vi "robot_focus.vi"(7 "Robot_connection":refnum<k5>, 8 "rotation_parameters":T4={"circle_radius (mm)"=6.5, "total_circle_angle (deg)"=0.0, "circle number of points"=18}, 9 "focus_parameters":T3={"Robot_vel"=0.3, "Robot_acc"=0.1, "Z-tolerance (mm)"=0.2, "Angle tolerance (deg)"=1.0, "n_frames"=1, "frame_width"=500}, 10 "Buttons":T2, 11 "img":u8[][](array[numeric])) -> (0 "wait_frames":dbl, 1 "indicators":T1, 2 "apply_config":bool, 3 "Fast_axis":bool)   [LabVIEW 2021]
panel:
  out "img_size_2":dbl
  out "img_size_1":dbl
  out "circle_state_indicator":dbl
  out "Close enough":bool
  out "angle":dbl
  in  "movement_wait_frames":dbl=5.0
  out "focus_routine_indicator":i8
  out "stepwise_angle":dbl
  in  "circle_state":i8=-2
  in  "freedrive_state":i8
  out "message_output":string
  in  "focus_routine_state":i8
  # "Robot Focus code"
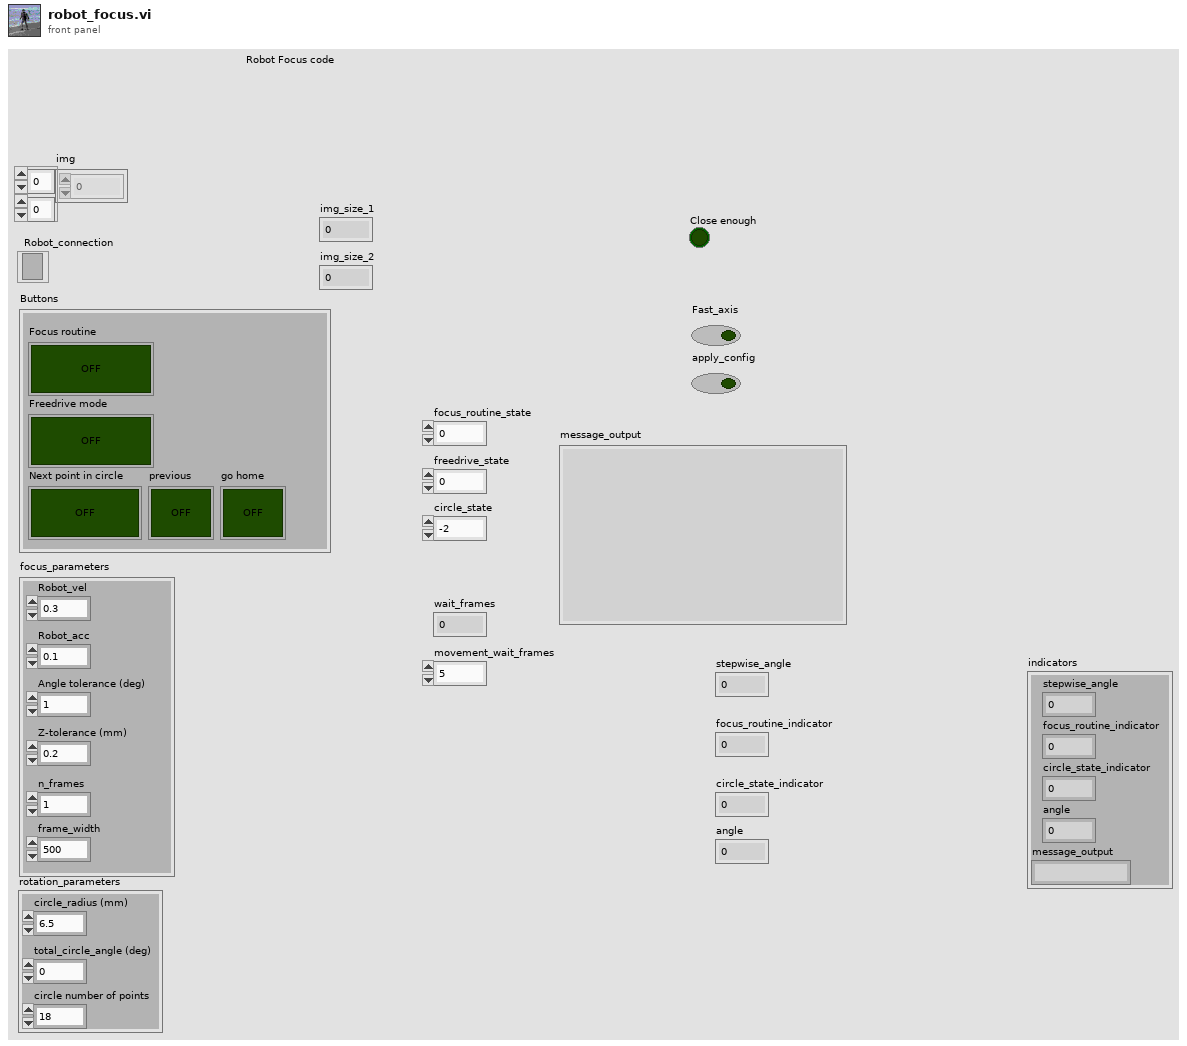
[diagram p1: front panel]
types:
  T1 = cluster{"stepwise_angle":dbl, "focus_routine_indicator":i8, "circle_state_indicator":dbl, "angle":dbl, "message_output":string}
  T2 = cluster{"Focus routine":bool, "Freedrive mode":bool, "Next point in circle":bool, "previous":bool, "go home":bool}
  T3 = cluster{"Robot_vel":dbl, "Robot_acc":dbl, "Z-tolerance (mm)":dbl, "Angle tolerance (deg)":dbl, "n_frames":i16, "frame_width":i16}
  T4 = cluster{"circle_radius (mm)":dbl, "total_circle_angle (deg)":dbl, "circle number of points":i8}
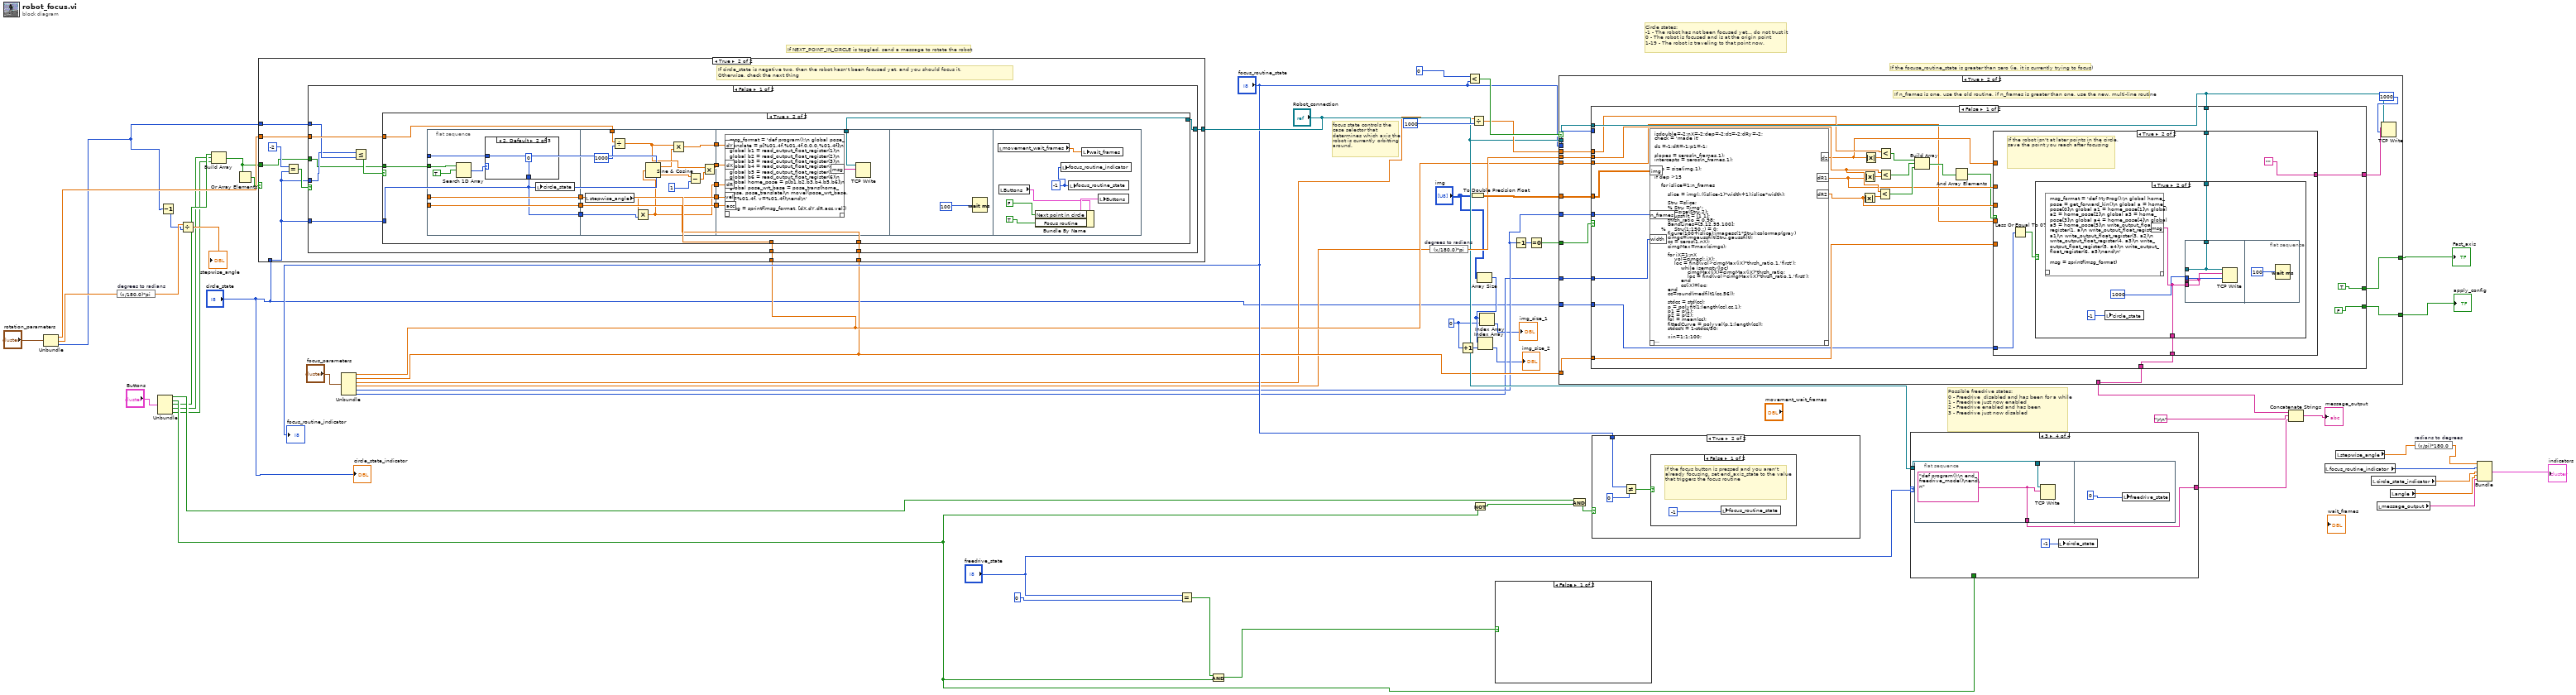
[diagram p0: block diagram]
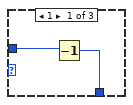
[diagram p4: hidden frame]
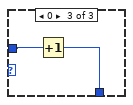
[diagram p5: hidden frame]
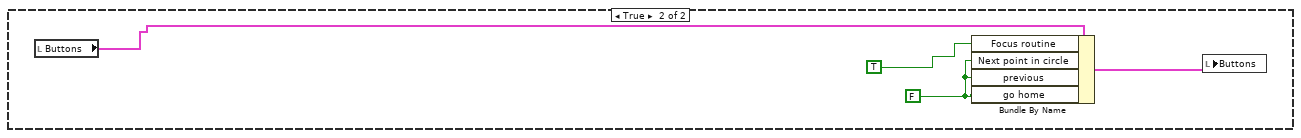
[diagram p6: hidden frame]
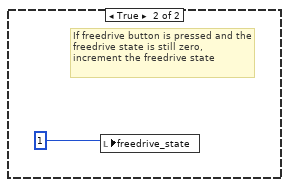
[diagram p7: hidden frame]
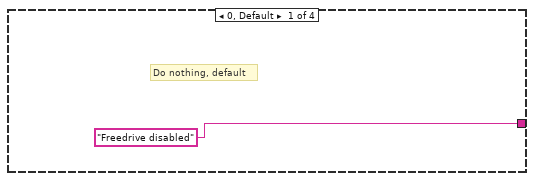
[diagram p8: hidden frame]
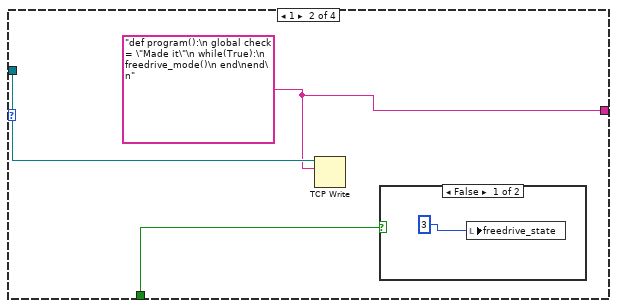
[diagram p9: hidden frame]
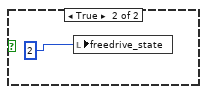
[diagram p10: hidden frame]
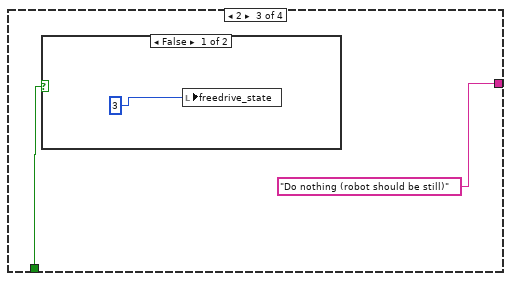
[diagram p11: hidden frame]
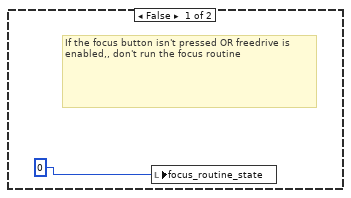
[diagram p13: hidden frame]
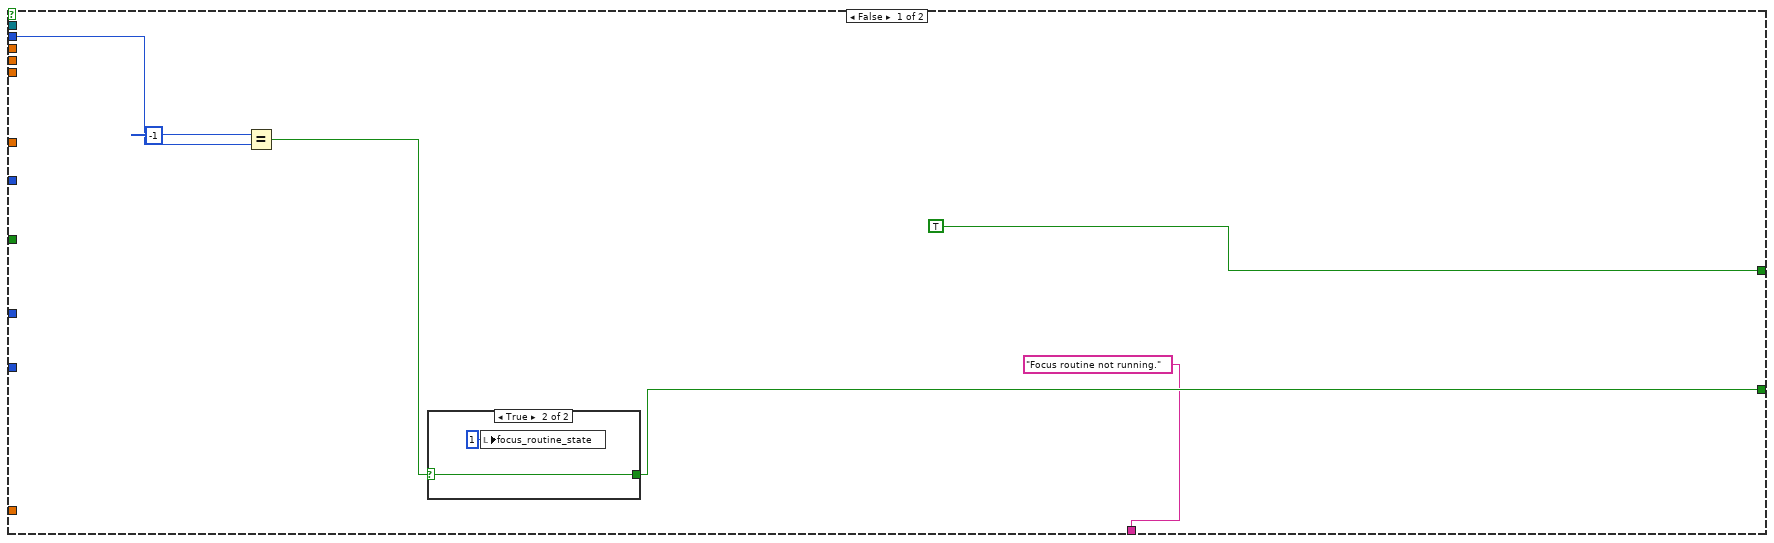
[diagram p15: hidden frame]
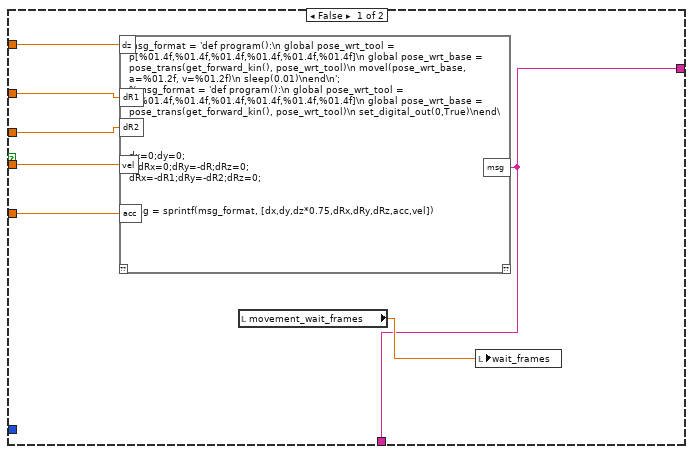
[diagram p17: hidden frame]
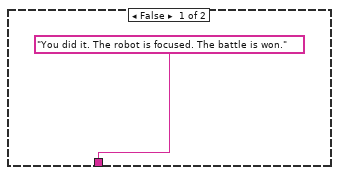
[diagram p18: hidden frame]
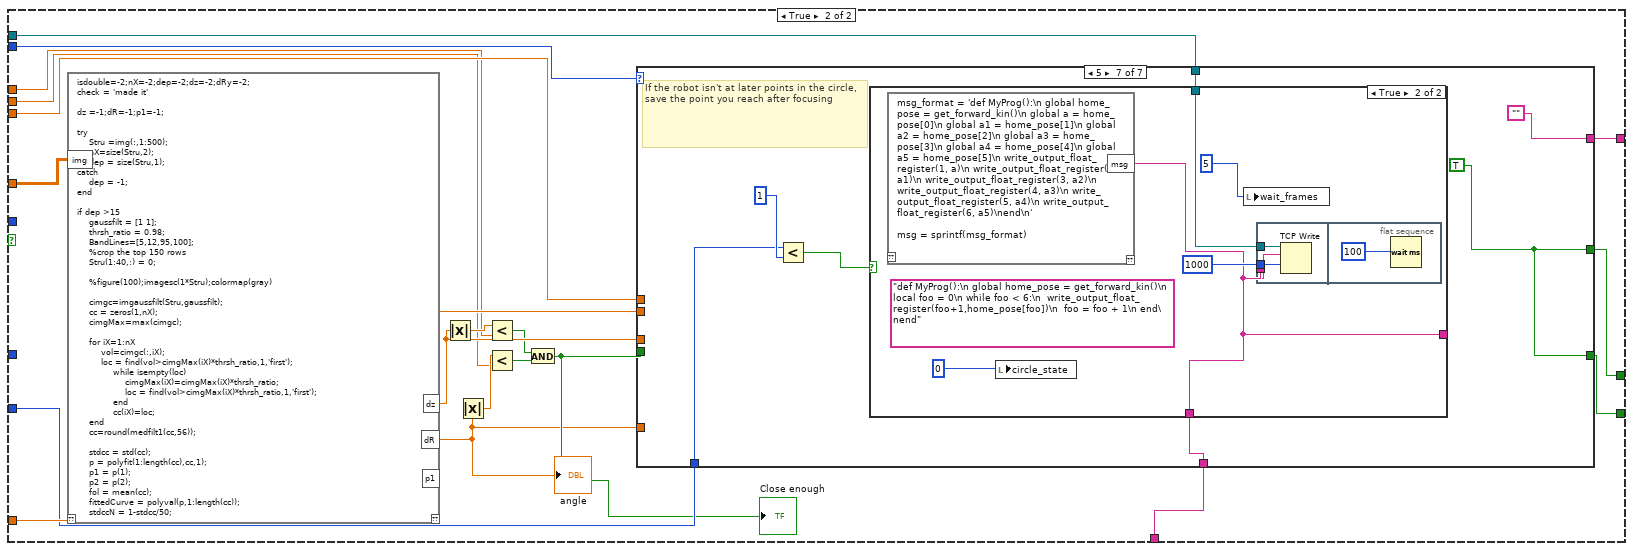
[diagram p19: hidden frame]
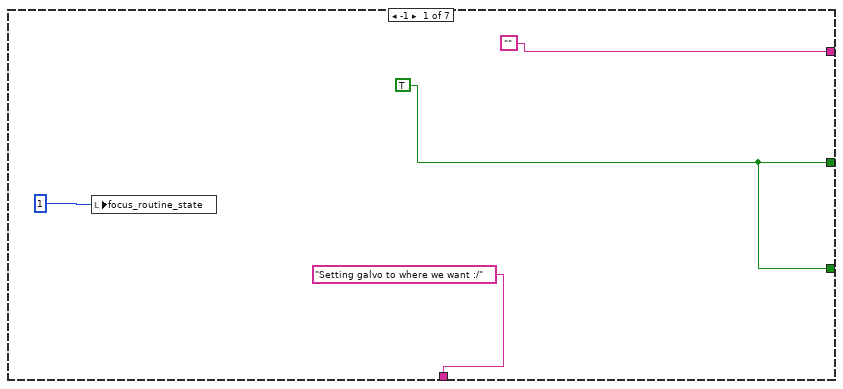
[diagram p20: hidden frame]
diagram:
  w15 = 0
  # "If NEXT_POINT_IN_CIRCLE is toggled, send a message to rotate the robot"
  # "If the focuse_routine_state is greater than zero (ie, it is currently trying to focus)"
  # "Circle states:\n-1 - The robot has not been focused yet... do not trust it\n0 - The robot is focused and is at the origin point\n1-19 - The robot is traveling to that point now."
  # "Possible freedrive states:\n0 - Freedrive  disabled and has been for a while\n1 - Freedrive just now enabled\n2 - Freedrive enabled and has been\n3 - Freedrive just now disabled"
  # "focus state controls the case selector that determines which axis the robot is currently orbitting around."
  n1 = Unbundle("rotation_parameters") -> ("circle_radius (mm)"=w34:dbl, "total_circle_angle (deg)"=w14:dbl, "circle number of points"=w10:i8)
  n2 = expression code="(x/180.0)*pi" "degrees to radians"(w14) -> (w13:dbl)
  n3 = Unbundle("Buttons") -> ("Focus routine"=w8:bool, "Freedrive mode"=w7:bool, "Next point in circle"=w5:bool, "previous"=w4:bool, "go home"=w3:bool)
  n4 = Decrement(x=w10) -> (x-1=w9:i8)
  n5 = Divide(x=w13, y=w9) -> (x/y=→"stepwise_angle":dbl)
  n6 = Build Array(w5, w4, w3) -> (w1:bool[])
  n7 = Or Array Elements(Boolean array=w1) -> (logical OR=w2:bool)
  n8 = Unbundle("focus_parameters") -> ("Robot_vel"=w32:dbl, "Robot_acc"=w31:dbl, "Z-tolerance (mm)"=w29:dbl, "Angle tolerance (deg)"=w30:dbl, "n_frames"=w27:i16, "frame_width"=w26:i16)
  n9 = case shown="True" w2 {
    tunnel: "circle_state" -> [_ w62]
    tunnel: w10 -> [_ w65]
    tunnel: w32 -> [_ w64]
    tunnel: w31 -> [_ w63]
    tunnel: w34 -> [_ w61]
    tunnel: "Robot_connection" -> [_ w60]
    tunnel: w1 -> [_ w59]
    frame False {
    }
    frame True {
      # "If circle_state is negative two, then the robot hasn't been focused yet, and you should focus it.\nOtherwise, check the next thing"
      n10 = Equal?(x=-2, y=w62) -> (x = y?=w66:bool)
      n11 = case shown="False" w66 {
        tunnel: w65 -> [w71 _]
        tunnel: w62 -> [w70 _]
        tunnel: w64 -> [w76 _]
        tunnel: w63 -> [w75 _]
        tunnel: w62 -> [w74 _]
        tunnel: w61 -> [w73 _]
        tunnel: w60 -> [w72 _]
        tunnel: w59 -> [w68 _]
        frame False {
          n12 = Less Or Equal?(x=w70, y=w71) -> (x <= y?=w69:bool)
          n13 = case shown="True" w69 {
            tunnel: w76 -> [_ w90]
            tunnel: w75 -> [_ w89]
            tunnel: w74 -> [_ w79]
            tunnel: w73 -> [_ w80]
            tunnel: w72 -> [_ w88]
            tunnel: w68 -> [_ w77]
            frame False {
            }
            frame True {
              n14 = flat-sequence {
                tunnel: w79 -> [w95]
                tunnel: w89 -> [w96]
                tunnel: w90 -> [w97]
                tunnel: [w97] -> w82
                tunnel: [w96] -> w81
                tunnel: [w91] -> w78
                tunnel: w77 -> [w94]
                tunnel: [w116] -> w87
                tunnel: [w115] -> w86
                tunnel: [w104] -> w85
                tunnel: [w105] -> w84
                tunnel: [w106] -> w83
                tunnel: w82 -> [w116]
                tunnel: w81 -> [w115]
                tunnel: w80 -> [w108]
                tunnel: w78 -> [w103]
                tunnel: w88 -> [w117]
                tunnel: w87 -> [w123]
                tunnel: w86 -> [w122]
                tunnel: w85 -> [w121]
                tunnel: w84 -> [w120]
                tunnel: w83 -> [w119]
                frame #0 {
                  n15 = Search 1D Array(1D array=w94, element=TRUE) -> (index of element=w92:i32)  [unwired: 1 in]
                  n16 = case shown="2, Default" w92 {
                    tunnel: w95 -> [w99 _ w102]
                    tunnel: [w98 0 w101] -> w91
                    frame 1 {
                      n17 = Decrement(x=w99) -> (x-1=w98:i8)
                    }
                    frame 2, Default {
                    }
                    frame 0 {
                      n18 = Increment(x=w102) -> (x+1=w101:i8)
                    }
                  }
                  n19 = local write "circle_state"(w91) -> ()
                }
                frame #1 {
                  n20 = local read "stepwise_angle"() -> (w110:dbl)
                  n21 = Divide(x=w108, y=1000) -> (x/y=w113:dbl)
                  n22 = Multiply(x=w110, y=w103) -> (x*y=w104:dbl)
                  n23 = Sine & Cosine(0:w104) -> (1:w111:dbl, 2:w114:dbl)
                  n24 = Multiply(x=w113, y=w111) -> (x*y=w105:dbl)
                  n25 = Subtract(x=w114, y=1) -> (x-y=w112:dbl)
                  n26 = Multiply(x=w113, y=w112) -> (x*y=w106:dbl)
                }
                frame #2 {
                  n27 = script code="msg_format = 'def program():\\n global pose_translate = p[%01.4f,%01.4f,0,0,0,%01.4f]\\n global b1 = read_output_float_register(1)\\n global b2 = read_output_float_register(2)\\n global b3 = read_output_float_register(3)\\n global b4 = read_output_float_register(4)\\n global b5 = read_output_float_register(5)\\n global b6 = read_output_float_register(6)\\n global home_pose = p[b1,b2,b3,b4,b5,b6]\\n global pose_wrt_base = pose_trans(home_pose, pose_translate)\\n movel(pose_wrt_base, a=%01.4f, v=%01.4f)\\nend\\n'\n\nmsg = sprintf(msg_format, [dX,dY,dR,acc,vel])"("dX"=w119, "dY"=w120, "dR"=w121, "vel"=w123, "acc"=w122) -> ("msg"=w118:string)  [unwired: 1 in, 1 out]
                  n28 = TCP Write(connection ID=w117, data in=w118) -> ()  [unwired: 2 in, 3 out]
                }
                frame #3 {
                  n29 = Wait (ms)(milliseconds to wait=100) -> ()  [unwired: 1 out]
                }
                frame #4 {
                  w130 = -1
                  n30 = local read "movement_wait_frames"() -> (w129:dbl)
                  n31 = local read "Buttons"() -> (w127:T2)
                  n32 = Bundle By Name(cluster=w127, "Next point in circle"=FALSE, "Focus routine"=TRUE) -> (w128:T2)
                  n33 = local write "focus_routine_indicator"(w130) -> ()
                  n34 = local write "focus_routine_state"(w130) -> ()
                  n35 = local write "wait_frames"(w129) -> ()
                  n36 = local write "Buttons"(w128) -> ()
                }
              }
            }
          }
        }
        frame True {
          w131 = FALSE
          n37 = local read "Buttons"() -> (w132:T2)
          n38 = Bundle By Name(cluster=w132, "Focus routine"=TRUE, "Next point in circle"=w131, "previous"=w131, "go home"=w131) -> (w133:T2)
          n39 = local write "Buttons"(w133) -> ()
        }
      }
    }
  }
  n40 = Equal?(x="freedrive_state", y=0) -> (x = y?=w43:bool)
  n41 = And(x=w43, y=w7) -> (x .and. y?=w42:bool)
  n42 = expression code="(x/180.0)*pi" "degrees to radians"(w30) -> (w55:dbl)
  n43 = Increment(x=w15) -> (x+1=w16:i32)
  n44 = Less?(x=0, y="focus_routine_state") -> (x < y?=w56:bool)
  n45 = To Double Precision Float(number="img") -> (double precision float=w58:dbl[][])
  n46 = Divide(x=w29, y=1000) -> (x/y=w52:dbl)
  n47 = Not(x=w7) -> (.not. x?=w49:bool)
  n48 = Array Size(array="img") -> (size(s)=w18:i32[])
  n49 = Index Array(array=w18, index=w16) -> (element=→"img_size_2":i32)
  n50 = Index Array(array=w18, index=w15) -> (element=→"img_size_1":i32)
  n51 = case shown="False" w42 {
    frame False {
    }
    frame True {
      # "If freedrive button is pressed and the freedrive state is still zero, increment the freedrive state"
      n52 = local write "freedrive_state"(1) -> ()
    }
  }
  n53 = Decrement(x=w27) -> (x-1=w37:i16)
  n54 = Equal To 0?(x=w37) -> (x = 0?=w36:bool)
  n55 = case shown="True" w56 {
    tunnel: w58 -> [_ w160]
    tunnel: "focus_routine_state" -> [w140 w159]
    tunnel: w32 -> [_ w158]
    tunnel: w31 -> [_ w157]
    tunnel: w52 -> [_ w156]
    tunnel: w55 -> [_ w155]
    tunnel: "Robot_connection" -> [_ w145]
    tunnel: [TRUE w152] -> w54
    tunnel: [w137 w151] -> w51
    tunnel: ["Focus routine not running." w150] -> w48
    tunnel: "circle_state" -> [_ w149]
    tunnel: w36 -> [_ w148]
    tunnel: w26 -> [_ w147]
    tunnel: w27 -> [_ w146]
    frame False {
      n56 = Equal?(x=-1, y=w140) -> (x = y?=w139:bool)
      n57 = case shown="True" w139 {
        selector: w139 -> [w142 w144]
        tunnel: [w142 w144] -> w137
        frame False {
        }
        frame True {
          n58 = local write "focus_routine_state"(1) -> ()
        }
      }
    }
    frame True {
      # "If n_frames is one, use the old routine, if n_frames is greater than one, use the new, multi-line routine"
      n59 = case shown="False" w148 {
        tunnel: w160 -> [w184 w224]
        tunnel: w159 -> [_ w223]
        tunnel: w158 -> [w168 w222]
        tunnel: w157 -> [w169 w221]
        tunnel: w156 -> [w180 w217]
        tunnel: w155 -> [w176 w216]
        tunnel: [w164 w213] -> w154
        tunnel: [TRUE w212] -> w152
        tunnel: [FALSE w211] -> w151
        tunnel: [w161 w210] -> w150
        tunnel: w149 -> [w162 w209]
        tunnel: w145 -> [_ w207]
        tunnel: w147 -> [w183 _]
        tunnel: w146 -> [w182 _]
        tunnel: w145 -> [w163 _]
        frame False {
          n60 = script code="isdouble=-2;nX=-2;dep=-2;dz=-2;dRy=-2;\ncheck = 'made it'\n\ndz =-1;dR=-1;p1=-1;\n\nslopes = zeros(n_frames,1);\nintercepts = zeros(n_frames,1);\n\ndep = size(img,1);\n    \nif dep >15\n    \n    for islice=1:n_frames\n\n        slice = img(:,((islice-1)*width+1):islice*width);\n        \n        Stru =slice;\n        % Stru =img';\n        nX=size(Stru,2);\n        gaussfilt = [1 1];\n        thrsh_ratio = 0.98;\n        BandLines=[5,12,95,100];\n    %     Stru(1:150,:) = 0;\n        figure(100+islice);imagesc(1*Stru);colormap(gray)\n        cimgc=imgaussfilt(Stru,gaussfilt);\n        cc = zeros(1,nX);\n        cimgMax=max(cimgc);\n    \n        for iX=1:nX\n            vol=cimgc(:,iX);\n            loc = find(vol>cimgMax(iX)*thrsh_ratio,1,'first');\n                while isempty(loc)\n                    cimgMax(iX)=cimgMax(iX)*thrsh_ratio;\n                    loc = find(vol>cimgMax(iX)*thrsh_ratio,1,'first');\n                end\n                cc(iX)=loc;\n        end\n        cc=round(medfilt1(cc,56));\n    \n        stdcc = std(cc);\n        p = polyfit(1:length(cc),cc,1);\n        p1 = p(1);\n        p2 = p(2);\n        fol = mean(cc);\n        fittedCurve = polyval(p,1:length(cc));\n        stdccN = 1-stdcc/50;\n    \n        xin=1:1:100;\n    \n        hold on; plot(cc, 'r')\n        hold on; plot(fittedCurve, 'b')\n    \n        angle_output = 9.65 * atan(p1);\n        output_2 = fol / 51.2;\n    \n        slope = p1;\n        intercept = fol;\n\n        slopes(islice) = slope;\n        intercepts(islice) = intercept;\n    end\n%\n\nend\n\nr1_slope = mean(slopes);\nr1_intercept = mean(intercepts);\nr2_slope = polyfit(round(linspace(1,500,3)),intercepts,1);\nr2_slope = r2_slope(1);\n\n\nr1_slope\nr1_intercept\nr2_slope\n\nangle_output = 9.65 * atan(p1);\noutput_2 = fol / 51.2;\n\ndz=(r1_intercept-210)/150/1000 * 1.2;\ndR1=atan(r1_slope)*0.9\ndR2=atan(r2_slope)*0.9"("img"=w184, "n_frames"=w182, "width"=w183) -> ("dz"=w172:dbl, "dR1"=w171:dbl, "dR2"=w170:dbl)  [unwired: 1 in, 1 out]
          n61 = Absolute Value(x=w170) -> (abs(x)=w178:dbl)
          n62 = Absolute Value(x=w171) -> (abs(x)=w177:dbl)
          n63 = Absolute Value(x=w172) -> (abs(x)=w181:dbl)
          n64 = Less?(x=w176, y=w178) -> (x < y?=w174:bool)
          n65 = Less?(x=w180, y=w181) -> (x < y?=w179:bool)
          n66 = Less?(x=w176, y=w177) -> (x < y?=w175:bool)
          n67 = Build Array(w179, w175, w174) -> (w173:bool[])
          n68 = And Array Elements(Boolean array=w173) -> (logical AND=w167:bool)
          n69 = case shown="True" w167 {
            tunnel: w172 -> [w191 _]
            tunnel: w171 -> [w190 _]
            tunnel: w170 -> [w189 _]
            tunnel: w169 -> [w188 _]
            tunnel: w168 -> [w187 _]
            tunnel: [w185 ""] -> w164
            tunnel: w163 -> [_ w195]
            tunnel: w162 -> [_ w193]
            tunnel: [w185 w192] -> w161
            frame False {
              n70 = script code="msg_format = 'def program():\\n global pose_wrt_tool = p[%01.4f,%01.4f,%01.4f,%01.4f,%01.4f,%01.4f]\\n global pose_wrt_base = pose_trans(get_forward_kin(), pose_wrt_tool)\\n movel(pose_wrt_base, a=%01.2f, v=%01.2f)\\n sleep(0.01)\\nend\\n';\n%msg_format = 'def program():\\n global pose_wrt_tool = p[%01.4f,%01.4f,%01.4f,%01.4f,%01.4f,%01.4f]\\n global pose_wrt_base = pose_trans(get_forward_kin(), pose_wrt_tool)\\n set_digital_out(0,True)\\nend\\n';\n\n\ndx=0;dy=0;\n%dRx=0;dRy=-dR;dRz=0;\ndRx=-dR1;dRy=-dR2;dRz=0;\n\n\nmsg = sprintf(msg_format, [dx,dy,dz*0.75,dRx,dRy,dRz,acc,vel])"("dz"=w191, "dR1"=w190, "vel"=w187, "acc"=w188, "dR2"=w189) -> ("msg"=w185:string)  [unwired: 1 in, 1 out]
              n71 = local read "movement_wait_frames"() -> (w186:dbl)
              n72 = local write "wait_frames"(w186) -> ()
            }
            frame True {
              # "If the robot isn't at later points in the circle, save the point you reach after focusing"
              n73 = Less Or Equal To 0?(x=w193) -> (x <= 0?=w194:bool)
              n74 = case shown="True" w194 {
                tunnel: w195 -> [_ w201]
                tunnel: ["You did it. The robot is focused. The battle is won." w198] -> w192
                frame False {
                }
                frame True {
                  n75 = script code="msg_format = 'def MyProg():\\n global home_pose = get_forward_kin()\\n global a = home_pose[0]\\n global a1 = home_pose[1]\\n global a2 = home_pose[2]\\n global a3 = home_pose[3]\\n global a4 = home_pose[4]\\n global a5 = home_pose[5]\\n write_output_float_register(1, a)\\n write_output_float_register(2, a1)\\n write_output_float_register(3, a2)\\n write_output_float_register(4, a3)\\n write_output_float_register(5, a4)\\n write_output_float_register(6, a5)\\nend\\n'\n\nmsg = sprintf(msg_format)"() -> ("msg"=w198:string)  [unwired: 1 in, 1 out]
                  n76 = local write "circle_state"(-1) -> ()
                  n77 = flat-sequence {
                    tunnel: [w202] -> _
                    tunnel: [w203] -> _
                    tunnel: 1000 -> [w204]
                    tunnel: w198 -> [w203]
                    tunnel: w201 -> [w202]
                    frame #0 {
                      n78 = TCP Write(connection ID=w202, data in=w203, 9:w204) -> ()  [unwired: 1 in, 3 out]
                    }
                    frame #1 {
                      n79 = Wait (ms)(milliseconds to wait=100) -> ()  [unwired: 1 out]
                    }
                  }
                }
              }
            }
          }
        }
        frame True {
          n80 = script code="isdouble=-2;nX=-2;dep=-2;dz=-2;dRy=-2;\ncheck = 'made it'\n\ndz =-1;dR=-1;p1=-1;\n\ntry\n    Stru =img(:,1:500);\n    nX=size(Stru,2);\n    dep = size(Stru,1);\ncatch\n    dep = -1;\nend\n    \nif dep >15\n    gaussfilt = [1 1];\n    thrsh_ratio = 0.98;\n    BandLines=[5,12,95,100];\n    %crop the top 150 rows\n    Stru(1:40,:) = 0;\n\n    %figure(100);imagesc(1*Stru);colormap(gray)\n    \n    cimgc=imgaussfilt(Stru,gaussfilt);\n    cc = zeros(1,nX);\n    cimgMax=max(cimgc);\n\n    for iX=1:nX\n        vol=cimgc(:,iX);\n        loc = find(vol>cimgMax(iX)*thrsh_ratio,1,'first');\n            while isempty(loc)\n                cimgMax(iX)=cimgMax(iX)*thrsh_ratio;\n                loc = find(vol>cimgMax(iX)*thrsh_ratio,1,'first');\n            end\n            cc(iX)=loc;\n    end\n    cc=round(medfilt1(cc,56));\n\n    stdcc = std(cc);\n    p = polyfit(1:length(cc),cc,1);\n    p1 = p(1);\n    p2 = p(2);\n    fol = mean(cc);\n    fittedCurve = polyval(p,1:length(cc));\n    stdccN = 1-stdcc/50;\n\n    xin=1:1:100;\n\n    %hold on; plot(cc, 'r')\n    %hold on; plot(fittedCurve, 'b')\n\n    angle_output = 9.65 * atan(p1);\n    output_2 = fol / 51.2;\n    dx=0;dy=0;dz=(fol-210)/150/1000 * 1.2;\n    %dRx=0;dRy=atan(p1)*0.2913;dRz=0;\n    dR=atan(p1)*0.9\n% \nend"("img"=w224) -> ("dz"=w220:dbl, "dR"=w206:dbl)  [unwired: 1 in, 2 out]
          "angle" <- w206
          n81 = Absolute Value(x=w220) -> (abs(x)=w218:dbl)
          n82 = Absolute Value(x=w206) -> (abs(x)=w219:dbl)
          n83 = Less?(x=w218, y=w217) -> (x < y?=w215:bool)
          n84 = Less?(x=w219, y=w216) -> (x < y?=w214:bool)
          n85 = And(x=w215, y=w214) -> (x .and. y?=w208:bool)
          "Close enough" <- w208
          n86 = case shown="5" w223 {
            tunnel: w220 -> [_ _ w240 w262 _ _ _]
            tunnel: w206 -> [_ _ w239 w261 _ _ _]
            tunnel: w222 -> [_ _ w238 w259 _ _ _]
            tunnel: w221 -> [_ _ w237 w260 _ _ _]
            tunnel: w208 -> [_ _ w236 w257 w281 w286 _]
            tunnel: ["" w230 w235 w258 "" "" ""] -> w213
            tunnel: [w228 TRUE w233 w255 TRUE w287 w297] -> w212
            tunnel: [w228 FALSE w234 w256 FALSE w287 w297] -> w211
            tunnel: ["Setting galvo to where we want :/" w230 w232 w254 "Just resolved axis 2, checking axis 1..." "Just resolved axis 1, checking axis 2..." w293] -> w210
            tunnel: w209 -> [_ _ _ _ _ _ w295]
            tunnel: w207 -> [_ _ _ _ _ _ w291]
            frame -1 {
              w228 = TRUE
              n87 = local write "focus_routine_state"(1) -> ()
            }
            frame 0, Default {
              w230 = "Focus routine not running (should be impossible, is inside another check against this) "
            }
            frame 1 {
              # "While this axis is actively focusing, the fast_axis is True, and the config shouldn't change.\nOnce this axis is focused, the fast_axis value should be False and the config /should/ change"
              n88 = case shown="False" w236 {
                tunnel: w240 -> [w248 _]
                tunnel: w239 -> [w247 _]
                tunnel: w238 -> [w246 _]
                tunnel: w237 -> [w245 _]
                tunnel: [w242 ""] -> w235
                tunnel: [FALSE TRUE] -> w234
                tunnel: [TRUE FALSE] -> w233
                tunnel: [w242 "Just resolved axis 1"] -> w232
                frame False {
                  # "Still focusing"
                  n89 = script code="msg_format = 'def program():\\n global pose_wrt_tool = p[%01.4f,%01.4f,%01.4f,%01.4f,%01.4f,%01.4f]\\n global pose_wrt_base = pose_trans(get_forward_kin(), pose_wrt_tool)\\n movel(pose_wrt_base, a=%01.2f, v=%01.2f)\\n sleep(0.01)\\nend\\n';\n%msg_format = 'def program():\\n global pose_wrt_tool = p[%01.4f,%01.4f,%01.4f,%01.4f,%01.4f,%01.4f]\\n global pose_wrt_base = pose_trans(get_forward_kin(), pose_wrt_tool)\\n set_digital_out(0,True)\\nend\\n';\n\n\ndx=0;dy=0;\n%dRx=0;dRy=-dR;dRz=0;\ndRx=-dR;dRy=0;dRz=0;\n\n\nmsg = sprintf(msg_format, [dx,dy,dz*0.75,dRx,dRy,dRz,acc,vel])"("dz"=w248, "dR"=w247, "vel"=w246, "acc"=w245) -> ("msg"=w242:string)  [unwired: 1 in, 1 out]
                  n90 = local read "movement_wait_frames"() -> (w241:dbl)
                  n91 = local write "wait_frames"(w241) -> ()
                }
                frame True {
                  n92 = local write "focus_routine_state"(4) -> ()
                }
              }
            }
            frame 2 {
              # "While this axis is actively focusing, the fast_axis is False, and the config shouldn't change.\nOnce this axis is focused, the fast_axis value should be True and the config /should/ change"
              n93 = case shown="False" w257 {
                tunnel: w262 -> [w270 _]
                tunnel: w261 -> [w269 _]
                tunnel: w260 -> [w268 _]
                tunnel: w259 -> [w267 _]
                tunnel: [w264 ""] -> w258
                tunnel: [FALSE TRUE] -> w256
                tunnel: [FALSE TRUE] -> w255
                tunnel: [w264 "Just resolved axis 2"] -> w254
                frame False {
                  n94 = script code="msg_format = 'def program():\\n global pose_wrt_tool = p[%01.4f,%01.4f,%01.4f,%01.4f,%01.4f,%01.4f]\\n global pose_wrt_base = pose_trans(get_forward_kin(), pose_wrt_tool)\\n movel(pose_wrt_base, a=%01.2f, v=%01.2f)\\n sleep(0.01)\\nend\\n';\n%msg_format = 'def program():\\n global pose_wrt_tool = p[%01.4f,%01.4f,%01.4f,%01.4f,%01.4f,%01.4f]\\n global pose_wrt_base = pose_trans(get_forward_kin(), pose_wrt_tool)\\n freedrive_mode()\\nend\\n';\n\ndx=0;dy=0;\n%dRx=-dR;dRy=0;dRz=0;\ndRx=0;dRy=-dR;dRz=0;\n\nmsg = sprintf(msg_format, [dx,dy,dz*0.75,dRx,dRy,dRz,acc,vel])"("dz"=w270, "dR"=w269, "acc"=w268, "vel"=w267) -> ("msg"=w264:string)  [unwired: 1 in, 1 out]
                  n95 = local read "movement_wait_frames"() -> (w263:dbl)
                  n96 = local write "wait_frames"(w263) -> ()
                }
                frame True {
                  n97 = local write "focus_routine_state"(3) -> ()
                }
              }
            }
            frame 3 {
              # "This is back to the original axis but we're checking whether or not it lines up... If it does line up we're done and go to state 5, and if it doesn't we need to go to state 1 and make adjustments again, but either way the fast axis value should stay the same as it was previously"
              n98 = case shown="True" w281 {
                tunnel: [1 5] -> w280
                frame False {
                }
                frame True {
                }
              }
              n99 = local write "focus_routine_state"(w280) -> ()
            }
            frame 4 {
              w287 = FALSE
              n100 = case shown="True" w286 {
                tunnel: [2 2] -> w288
                frame False {
                }
                frame True {
                }
              }
              n101 = local write "focus_routine_state"(w288) -> ()
            }
            frame 5 {
              w297 = TRUE
              # "If the robot isn't at later points in the circle, save the point you reach after focusing"
              n102 = Less?(x=w295, y=1) -> (x < y?=w294:bool)
              n103 = case shown="True" w294 {
                tunnel: ["" w300] -> _
                tunnel: ["Focus reached! Exitting..." w300] -> w293
                tunnel: w291 -> [_ w302]
                frame False {
                }
                frame True {
                  (unwired) "def MyProg():\n global home_pose = get_forward_kin()\n local foo = 0\n while foo < 6:\n  write_output_float_register(foo+1,home_pose[foo])\n  foo = foo + 1\n end\nend"
                  n104 = script code="msg_format = 'def MyProg():\\n global home_pose = get_forward_kin()\\n global a = home_pose[0]\\n global a1 = home_pose[1]\\n global a2 = home_pose[2]\\n global a3 = home_pose[3]\\n global a4 = home_pose[4]\\n global a5 = home_pose[5]\\n write_output_float_register(1, a)\\n write_output_float_register(2, a1)\\n write_output_float_register(3, a2)\\n write_output_float_register(4, a3)\\n write_output_float_register(5, a4)\\n write_output_float_register(6, a5)\\nend\\n'\n\nmsg = sprintf(msg_format)"() -> ("msg"=w300:string)  [unwired: 1 in, 1 out]
                  n105 = local write "circle_state"(0) -> ()
                  n106 = local write "wait_frames"(5) -> ()
                  n107 = flat-sequence {
                    tunnel: w302 -> [w307]
                    tunnel: w300 -> [w306]
                    tunnel: 1000 -> [w305]
                    frame #0 {
                      n108 = TCP Write(connection ID=w307, data in=w306, 9:w305) -> ()  [unwired: 1 in, 3 out]
                    }
                    frame #1 {
                      n109 = Wait (ms)(milliseconds to wait=100) -> ()  [unwired: 1 out]
                    }
                  }
                }
              }
            }
          }
        }
      }
      n110 = TCP Write(connection ID=w145, data in=w154, 9:1000) -> ()  [unwired: 1 in, 3 out]
    }
  }
  "Fast_axis" <- w54
  "apply_config" <- w51
  n111 = And(x=w8, y=w49) -> (x .and. y?=w50:bool)
  n112 = case shown="True" w50 {
    tunnel: "focus_routine_state" -> [_ w312]
    frame False {
      # "If the focus button isn't pressed OR freedrive is enabled,, don't run the focus routine"
      n113 = local write "focus_routine_state"(0) -> ()
    }
    frame True {
      n114 = Not Equal?(x=w312, y=0) -> (x != y?=w310:bool)
      n115 = case shown="False" w310 {
        frame False {
          # "If the focus button is pressed and you aren't already focusing, set end_axis_state to the value that triggers the focus routine"
          n116 = local write "focus_routine_state"(-1) -> ()
        }
        frame True {
          # "If the focus button is pressed but you're already focusing, do nothing"
        }
      }
    }
  }
  n117 = case shown="3" "freedrive_state" {
    tunnel: "Robot_connection" -> [_ w317 _ w325]
    tunnel: ["Freedrive disabled" w315 "Do nothing (robot should be still)" w324] -> w45
    tunnel: w7 -> [_ w316 w320 _]
    frame 0, Default {
      # "Do nothing, default"
    }
    frame 1 {
      w315 = "def program():\n global check = \"Made it\"\n while(True):\n  freedrive_mode()\n end\nend\n"
      n118 = TCP Write(connection ID=w317, data in=w315) -> ()  [unwired: 2 in, 3 out]
      n119 = case shown="False" w316 {
        frame False {
          n120 = local write "freedrive_state"(3) -> ()
        }
        frame True {
          n121 = local write "freedrive_state"(2) -> ()
        }
      }
    }
    frame 2 {
      n122 = case shown="False" w320 {
        frame False {
          n123 = local write "freedrive_state"(3) -> ()
        }
        frame True {
        }
      }
    }
    frame 3 {
      n124 = flat-sequence {
        tunnel: w325 -> [w327]
        tunnel: [w326] -> w324
        frame #0 {
          w326 = "def program():\n end_freedrive_mode()\nend\n"
          n125 = TCP Write(connection ID=w327, data in=w326) -> ()  [unwired: 2 in, 3 out]
        }
        frame #1 {
          n126 = local write "freedrive_state"(0) -> ()
        }
      }
      n127 = local write "circle_state"(-1) -> ()
    }
  }
  n128 = Concatenate Strings(w48, "\r\n", w45) -> (→"message_output":string)
  n129 = local read "focus_routine_indicator"() -> (w25:i8)
  n130 = local read "stepwise_angle"() -> (w12:dbl)
  n131 = local read "circle_state_indicator"() -> (w24:dbl)
  n132 = local read "message_output"() -> (w22:string)
  n133 = local read "angle"() -> (w23:dbl)
  n134 = expression code="(x/pi)*180.0" "radians to degrees"(w12) -> (w11:dbl)
  n135 = Bundle("stepwise_angle"=w11, "focus_routine_indicator"=w25, "circle_state_indicator"=w24, "angle"=w23, "message_output"=w22) -> (→"indicators":T1)  [unwired: 1 in]
  "focus_routine_indicator" <- "focus_routine_state"
  "circle_state_indicator" <- "circle_state"
